vi "MenuFind.vi"(1 "TagIn":string) -> (0 "Menu":string)   [LabVIEW 2014]
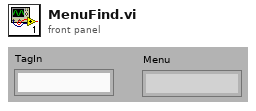
[diagram p1: front panel]
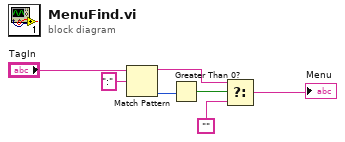
[diagram p0: block diagram]
diagram:
  n1 = Match Pattern(string="TagIn", regular expression=":" ("search string/char (-)")) -> (before substring=w1:string, offset past match=w5:i32)  [unwired: 1 in, 2 out]
  n2 = Greater Than 0?(x=w5) -> (x > 0?=w4:bool)
  n3 = Select(t=w1, s=w4, f="") -> (s? t:f=→"Menu":string)
